vi "Initialize Background UI.vi"(8 "error in":errorcluster, 9 "Reference In":variant, 11 "Inset in":refnum<class "Inset.lvclass">) -> (0 "error out":errorcluster, 1 "Image Control":T1, 3 "Inset out":refnum<class "Inset.lvclass">)   [LabVIEW 2019, in "Inset.lvclass"]
uses:
  Inset.lvclass
  BigMAQ/BigMAQ.lvclass
  <vilib>/vision/Image Controls.llb/IMAQ Image.ctl
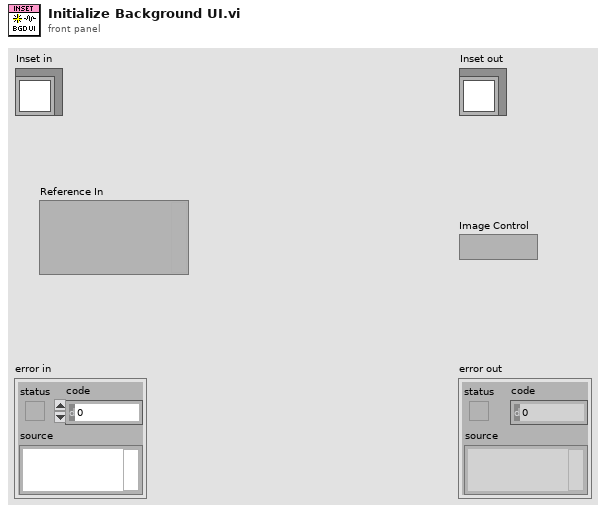
[diagram p1: front panel]
types:
  T1 = typedef "IMAQ Image.ctl" = refnum<image>
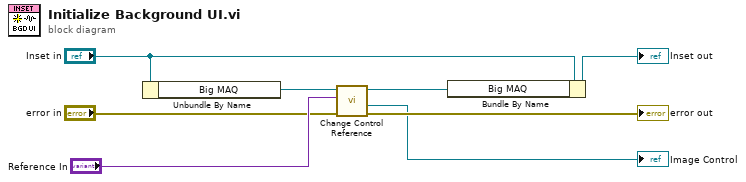
[diagram p0: block diagram]
diagram:
  n1 = Unbundle By Name("Inset in") -> ("Big MAQ"=w8:refnum<class "BigMAQ.lvclass">)
  n2 = call "Change Control Reference.vi"("error in"="error in", "Reference In"="Reference In", "BigMAQ in"=w8) -> ("error out"=→"error out":errorcluster, "Image Control"=→"Image Control":T1, "BigMAQ out"=w7:refnum<class "BigMAQ.lvclass">)  [unwired: 6 in]
  n3 = Bundle By Name(cluster="Inset in", "Big MAQ"=w7) -> (→"Inset out":refnum<class "Inset.lvclass">)
